vi "Clear Ball.vi"(11 "AI Manager in":refnum<class "AI Manager.lvclass">) -> (2 "Direction out":cluster{dbl, dbl}, 5 "Boost?":bool)   [LabVIEW 2021, in "AI Manager.lvclass"]
doc: "MIT Licence\nCopyright (c) 2024 David Grollier"
uses:
  AI Manager.lvclass
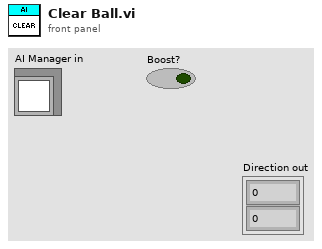
[diagram p1: front panel]
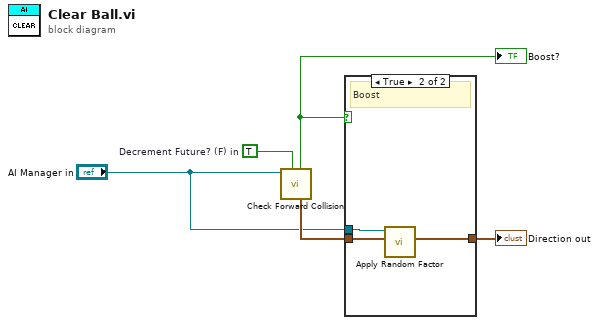
[diagram p0: block diagram]
diagram:
  w5 = TRUE  # Decrement Future? (F) in
  n1 = call "Check Forward Collision.vi"("Decrement Future? (F) in"=w5, "AI Manager in"="AI Manager in") -> ("Vector direction out"=w3:cluster{dbl, dbl}, "Collision?"=w4:bool)  [unwired: 6 in, 2 out]
  "Boost?" <- w4
  n2 = case shown="True" w4 {
    tunnel: w3 -> [w6 w9]
    tunnel: "AI Manager in" -> [_ w8]
    tunnel: [w6 w7] -> w1
    frame False {
      # "No boost"
    }
    frame True {
      # "Boost"
      n3 = call "Apply Random Factor.vi"("Velocity in"=w9, "AI Manager in"=w8) -> ("Adjusted Velocity out"=w7:cluster{dbl, dbl})  [unwired: 9 in]
    }
  }
  "Direction out" <- w1
